vi "Write Analogue.vi"(8 "error in (no error)":errorcluster, 10 "Boolean":bool, 11 "Sim PS in":refnum<class "Sim PS.lvclass">) -> (0 "error out":errorcluster, 3 "Sim PS out":refnum<class "Sim PS.lvclass">)   [LabVIEW 2021, in "Concrete.lvlib" / "Sim PS.lvclass"]
uses:
  Sim PS.lvclass
  Harware Abstraction/AnalogIO/Power Supply.lvclass
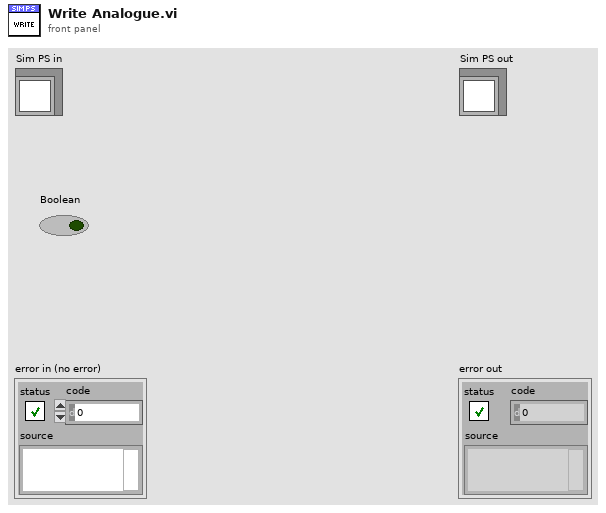
[diagram p1: front panel]
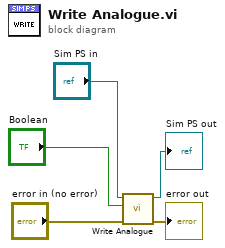
[diagram p0: block diagram]
diagram:
  n1 = call-parent "Write Analogue.vi"("error in (no error)"="error in (no error)", "Outbput"="Boolean", "PS in"="Sim PS in") -> ("error out"=→"error out":errorcluster, "PS out"=→"Sim PS out":refnum<class "Sim PS.lvclass">)  [unwired: 7 in]
